vi "Create.vi"(8 "error in (no error)":errorcluster, 9 "Calculation Period (ms)":u32=500, 10 "XNET Session":refnum<k21>, 11 "CANBus_Load_Calculator in":refnum<class "CANBus_Load_Calculator.lvclass">) -> (0 "error out":errorcluster, 3 "CANBus_Load_Calculator out":refnum<class "CANBus_Load_Calculator.lvclass">)   [LabVIEW 2018, in "NI-XNET Monitor Engine.lvlib" / "XNET-Bus-Load-Calculator.lvlib" / "CANBus_Load_Calculator.lvclass"]
uses:
  CANBus_Load_Calculator.lvclass
  <resource>/objmgr/xnet.rc
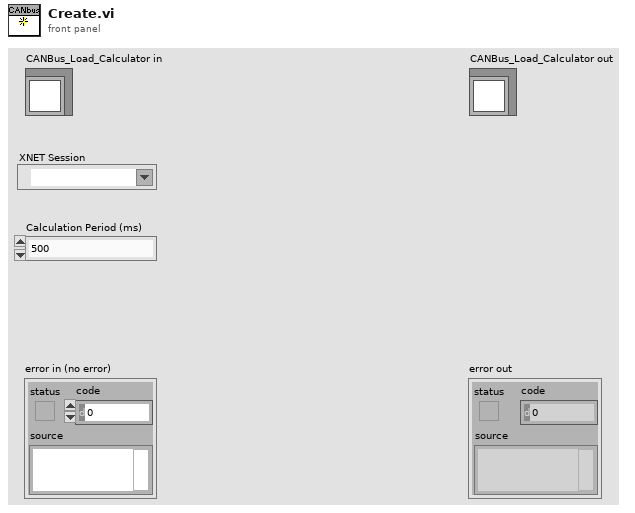
[diagram p1: front panel]
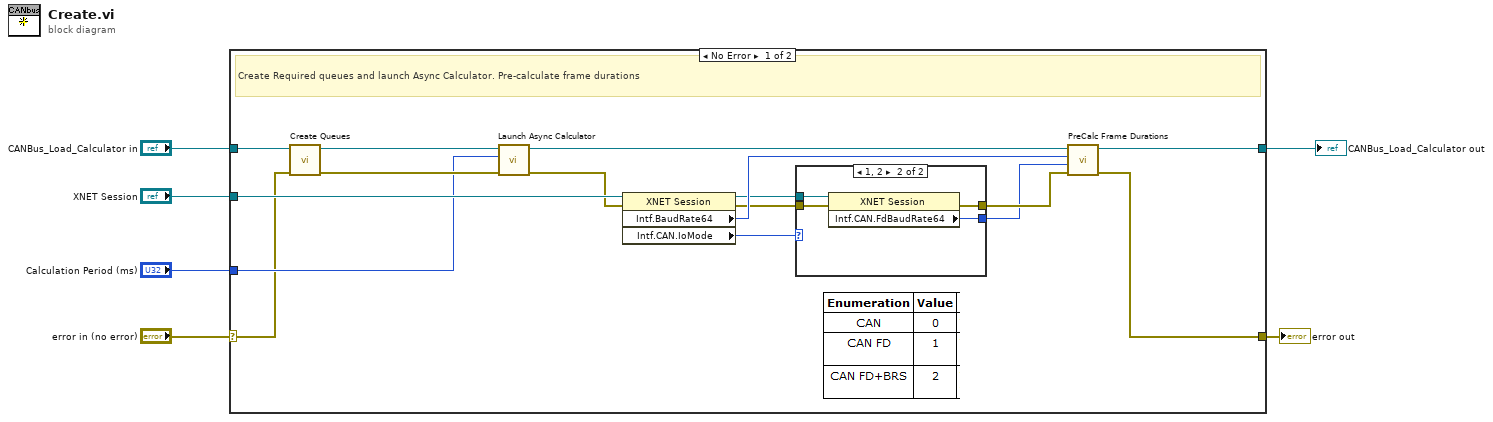
[diagram p0: block diagram]
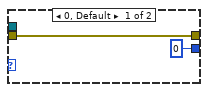
[diagram p2: hidden frame]
diagram:
  n1 = case shown="No Error" "error in (no error)" {
    selector: "error in (no error)" -> [w12 w29]
    tunnel: [w22 w30] -> w6
    tunnel: "Calculation Period (ms)" -> [w13 _]
    tunnel: "XNET Session" -> [w21 _]
    tunnel: "CANBus_Load_Calculator in" -> [w16 w30]
    tunnel: [w19 w29] -> w1
    frame No Error {
      # "Create Required queues and launch Async Calculator. Pre-calculate frame durations"
      n2 = call "Create Queues.vi"("error in (no error)"=w12, "GenBus_Load_Calculator in"=w16) -> ("error out"=w17:errorcluster, "GenBus_Load_Calculator out"=w18:refnum<class "CANBus_Load_Calculator.lvclass">)  [unwired: 8 in]
      n3 = call "Launch Async Calculator.vi"("error in (no error)"=w17, "Calculation Period (ms)"=w13, "Load Calculator in"=w18) -> ("error out"=w14:errorcluster, "Load Calculator out"=w15:refnum<class "CANBus_Load_Calculator.lvclass">)  [unwired: 7 in]
      n4 = property class="XNET Session"(reference=w21, error in=w14) -> (reference out=w11:refnum<k21>, error out=w10:errorcluster, "Intf.BaudRate64"=w20:u64, "Intf.CAN.IoMode"=w7:u32)
      n5 = case shown="1, 2" w7 {
        tunnel: w11 -> [_ w28]
        tunnel: w10 -> [w24 w27]
        tunnel: [w24 w26] -> w9
        tunnel: [u64 0 ("Intf.CAN.FdBaudRate64") w25] -> w8
        frame 0, Default {
        }
        frame 1, 2 {
          n6 = property class="XNET Session"(reference=w28, error in=w27) -> (error out=w26:errorcluster, "Intf.CAN.FdBaudRate64"=w25:u64)  [unwired: 1 out]
        }
      }
      n7 = call "PreCalc Frame Durations.vi"("error in (no error)"=w9, "FD Baud Rate"=w8, "Baud Rate"=w20, "CAN Bus Class In"=w15) -> ("error out"=w19:errorcluster, "CAN Bus Class Out"=w22:refnum<class "CANBus_Load_Calculator.lvclass">)  [unwired: 6 in]
    }
    frame Error {
    }
  }
  "error out" <- w1
  "CANBus_Load_Calculator out" <- w6
